vi "Render Template (Path).vi"(6 "Locals (None)":refnum<class "Value Tree.lvclass">, 8 "error in (no error)":errorcluster, 10 "Path":path, 11 "TemplateService in":refnum<class "TemplateService.lvclass">) -> (0 "error out":errorcluster, 2 "String":string, 3 "TemplateService out":refnum<class "TemplateService.lvclass">)   [LabVIEW 2020, in "HTTP Server.lvlib" / "TemplateService.lvclass"]
uses:
  TemplateService.lvclass
  Value Tree/Value Tree.lvclass
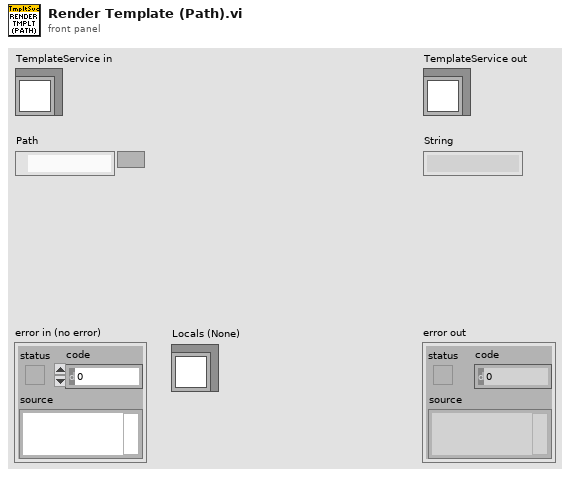
[diagram p1: front panel]
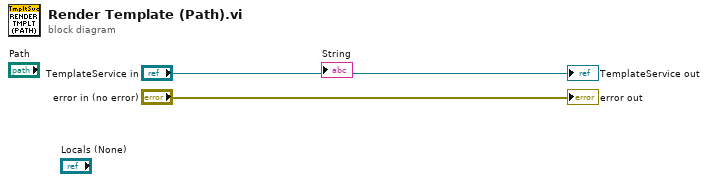
[diagram p0: block diagram]
diagram:
  "error out" <- "error in (no error)"
  "TemplateService out" <- "TemplateService in"
